vi "Read Histogram.vi"(8 "error in (no error)":errorcluster {"code" format="%.0x"}, 9 "Bin Range (0: 8 A)":i32(ring) items=["8 A", "0.0039 A"], 10 "Channel Name (1)":string="1", 11 "VISA resource name":refnum<visa-resource-name>) -> (0 "error out":errorcluster {"code" format="%.0x"}, 2 "Bin Data":dbl[](array[numeric]) format="%^.3e", 3 "VISA resource name out":refnum<visa-resource-name>)   [LabVIEW 2016, in "Agilent N6700 Series.lvlib"]
doc: "Reads and returns the bin data in the histogram.\n\n<b>Notes:</b>\n(1) This VI only applies to models N678xA SMU that have the Data Logger function installed.\n(2) This VI only applies to the N6705B and N6705C DC Power Analyzer."
uses:
  <instrlib>/Agilent N6700 Series/Agilent N6700 Series.lvlib
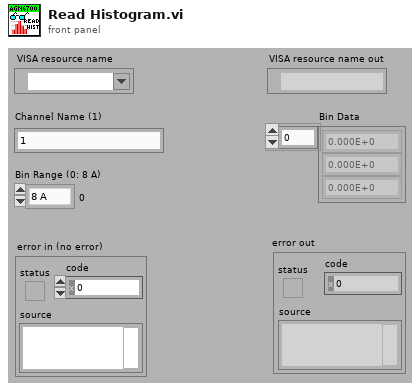
[diagram p1: front panel]
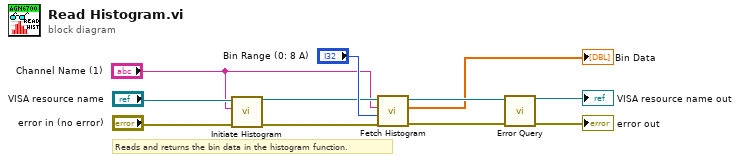
[diagram p0: block diagram]
diagram:
  # "Reads and returns the bin data in the histogram function."
  n1 = call <instrlib>:"Initiate Histogram.vi"("error in (no error)"="error in (no error)", "Channel Name (1)"="Channel Name (1)", "VISA resource name"="VISA resource name") -> ("error out"=w6:errorcluster, "VISA resource name out"=w5:refnum<visa-resource-name>)  [unwired: 7 in]
  n2 = call <instrlib>:"Fetch Histogram.vi"("error in (no error)"=w6, "Bin Range (0: 8A)"="Bin Range (0: 8 A)", "Channel Name (1)"="Channel Name (1)", "VISA resource name"=w5) -> ("error out"=w7:errorcluster, "Bin Data"=→"Bin Data":dbl[], "VISA resource name out"=w8:refnum<visa-resource-name>)  [unwired: 5 in]
  n3 = call <instrlib>:"Error Query.vi"("VISA resource name"=w8, "error in (no error)"=w7) -> ("VISA resource name out"=→"VISA resource name out":refnum<visa-resource-name>, "error out"=→"error out":errorcluster)  [unwired: 10 in, 2 out]
